vi "Write Sub Panel Coins.vi"(8 "error in (no error)":errorcluster, 10 "Sub Panel Coins":refnum<vi>, 11 "Actor_USD in":refnum<class "Actor_USD.lvclass">) -> (0 "error out":errorcluster, 3 "Actor_USD out":refnum<class "Actor_USD.lvclass">)   [LabVIEW 2019, in "Actor_USD.lvlib" / "Actor_USD.lvclass"]
uses:
  Actor_USD.lvclass
  Actor_USD.lvclass/Actor_USD.ctl
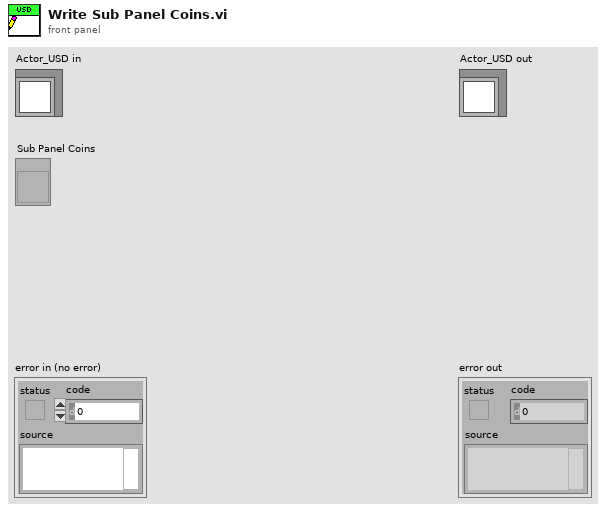
[diagram p1: front panel]
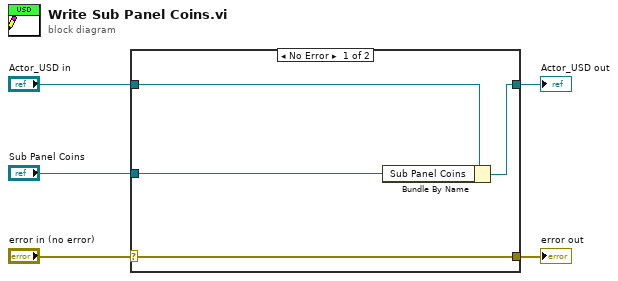
[diagram p0: block diagram]
diagram:
  n1 = case shown="No Error" "error in (no error)" {
    selector: "error in (no error)" -> [w9 w10]
    tunnel: [w9 w10] -> w4
    tunnel: [w7 w11] -> w2
    tunnel: "Actor_USD in" -> [w8 w11]
    tunnel: "Sub Panel Coins" -> [w6 _]
    frame No Error {
      n2 = Bundle By Name(cluster=w8, "Sub Panel Coins"=w6) -> (w7:refnum<class "Actor_USD.lvclass">)
    }
    frame Error {
    }
  }
  "error out" <- w4
  "Actor_USD out" <- w2
